vi "Compile Datalog Array sub_VI.vi"(0 "Loop Runtime (s)":dbl, 1 "Total Runtime (s)":dbl, 2 "Initialised Array":dbl[][](array[numeric]), 5 "Encoder Output":T3, 7 "X Axis Motor Params":T2, 9 "Y Axis Motor Params":T1, 11 "Coordinates Input":T5) -> (8 "Data Array":dbl[][](array[numeric]))   [LabVIEW 2017]
uses:
  Coords Input Cluster.ctl
  X-Y Manipulator/XY PID manual setpoint/Encoder Cluster.ctl
  <vilib>/myRIO/Common/Instrument Driver Framework/myRIO v1.0/Encoder/typedefs/Encoder Count Direction Enum.ctl
  X Axis Motor Cluster.ctl
  Y Axis Motor Cluster.ctl
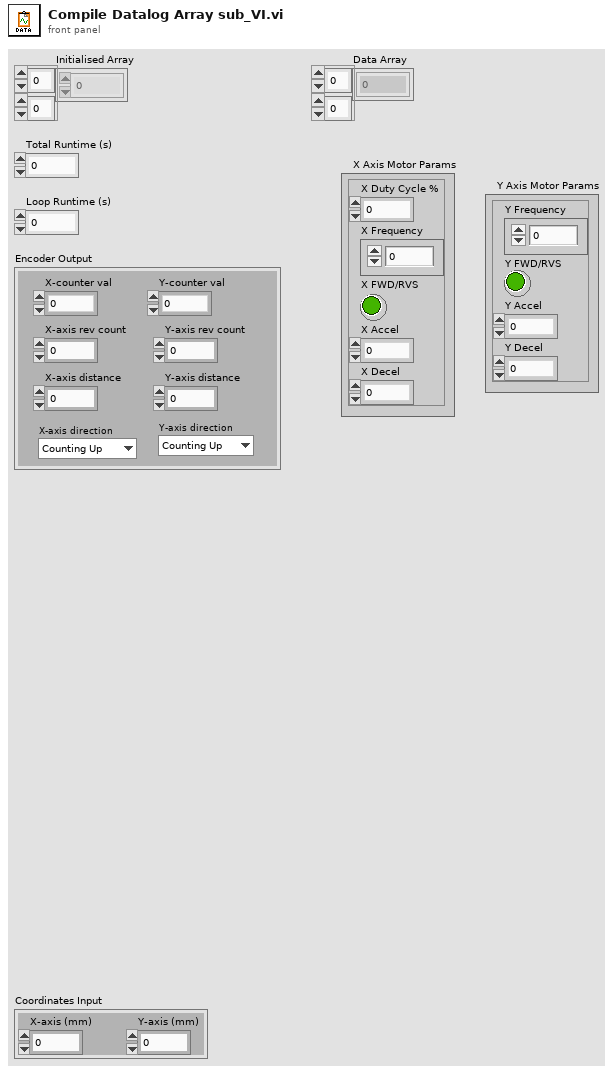
[diagram p1: front panel]
types:
  T1 = typedef "Y Axis Motor Cluster.ctl" = cluster{"Y Frequency":dbl, "Y FWD/RVS":bool, "Y Accel":dbl, "Y Decel":dbl}
  T2 = typedef "X Axis Motor Cluster.ctl" = cluster{"X Frequency":dbl, "X FWD/RVS":bool, "X Accel":dbl, "X Decel":dbl, "X Duty Cycle %":dbl}
  T3 = typedef "Encoder Cluster.ctl" = cluster{"Y-axis rev count":dbl, "Y-axis distance":dbl, "X-axis rev count":dbl, "X-axis distance":dbl, "Y-axis direction":T4, "X-axis direction":T4, "X-counter val":i32, "Y-counter val":i32}
  T4 = typedef "Encoder Count Direction Enum.ctl" = enum16{"Counting Up", "Counting Down"}
  T5 = typedef "Coords Input Cluster.ctl" = cluster{"X-axis (mm)":dbl, "Y-axis (mm)":dbl}
  T6 = cluster{"Total Runtime (s)":dbl, "Loop Runtime (s)":dbl, "X-axis distance":dbl, "X Duty Cycle %":dbl, "X Frequency":dbl, "Y-axis distance":dbl, "Y Frequency":dbl, "X Accel":dbl, "X Decel":dbl, "Y Accel":dbl, "Y Decel":dbl, "X-axis (mm)":dbl, "Y-axis (mm)":dbl, "Velocity (mm/s)":dbl, "Acceleration (mm/s^2)":dbl, "Velocity (mm/s)":dbl, "Acceleration (mm/s^2)":dbl}
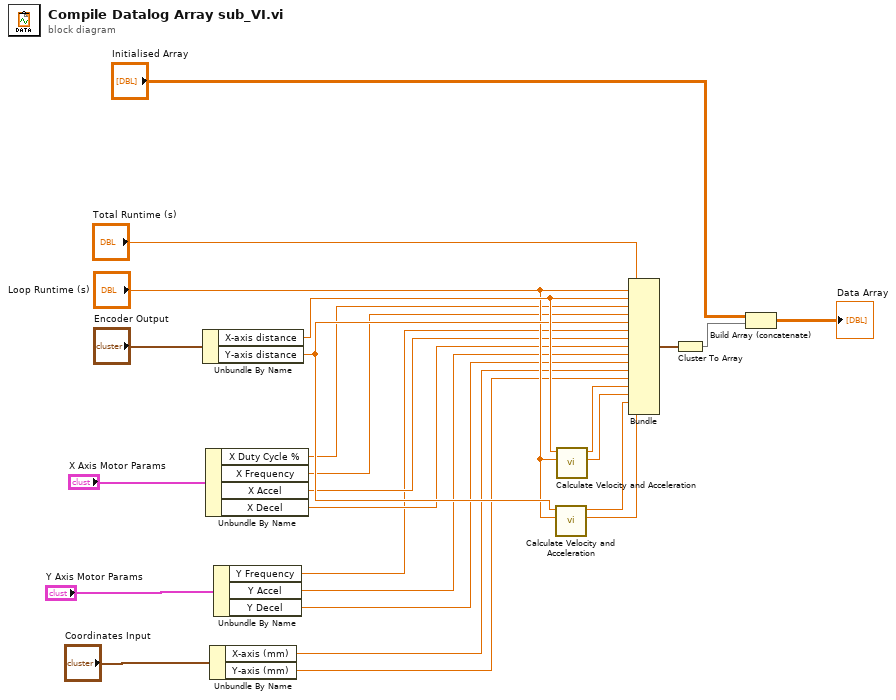
[diagram p0: block diagram]
diagram:
  n1 = Unbundle By Name("Encoder Output") -> ("X-axis distance"=w22:dbl, "Y-axis distance"=w21:dbl)
  n2 = Unbundle By Name("X Axis Motor Params") -> ("X Duty Cycle %"=w8:dbl, "X Frequency"=w9:dbl, "X Accel"=w11:dbl, "X Decel"=w12:dbl)
  n3 = Unbundle By Name("Coordinates Input") -> ("X-axis (mm)"=w16:dbl, "Y-axis (mm)"=w17:dbl)
  n4 = Unbundle By Name("Y Axis Motor Params") -> ("Y Frequency"=w10:dbl, "Y Accel"=w13:dbl, "Y Decel"=w14:dbl)
  n5 = call "Calculate Velocity and Acceleration.vi"("Loop Runtime (s)"="Loop Runtime (s)", "Displacement (mm)"=w21) -> ("Acceleration (mm/s^2)"=w24:dbl, "Velocity (mm/s)"=w23:dbl)  [unwired: 8 in]
  n6 = call "Calculate Velocity and Acceleration.vi"("Loop Runtime (s)"="Loop Runtime (s)", "Displacement (mm)"=w22) -> ("Acceleration (mm/s^2)"=w19:dbl, "Velocity (mm/s)"=w18:dbl)  [unwired: 8 in]
  n7 = Bundle("Total Runtime (s)"="Total Runtime (s)", "Loop Runtime (s)"="Loop Runtime (s)", "X-axis distance"=w22, "X Duty Cycle %"=w8, "X Frequency"=w9, "Y-axis distance"=w21, "Y Frequency"=w10, "X Accel"=w11, "X Decel"=w12, "Y Accel"=w13, "Y Decel"=w14, "X-axis (mm)"=w16, "Y-axis (mm)"=w17, "Velocity (mm/s)"=w18, "Acceleration (mm/s^2)"=w19, "Velocity (mm/s)"=w23, "Acceleration (mm/s^2)"=w24) -> (w4:T6)  [unwired: 1 in]
  n8 = Cluster To Array(cluster=w4) -> (array=w3:dbl[])
  n9 = Build Array (concatenate)("Initialised Array", w3) -> (→"Data Array":dbl[][])
